vi "Gen - Button Disable.vi"(6 "State":enum16{"Enable", "Disable", "Disable & Gray"}(ring), 8 "Error In":errorcluster, 11 "Ref in":refnum<vi>) -> (0 "Error Out":errorcluster)   [LabVIEW 2020]
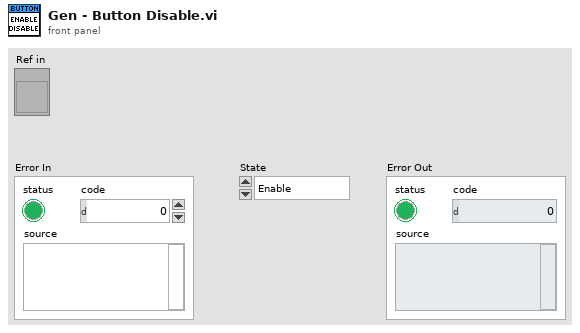
[diagram p1: front panel]
types:
  T1 = enum8{"Enabled", "Disabled", "Disabled and Grayed Out"}
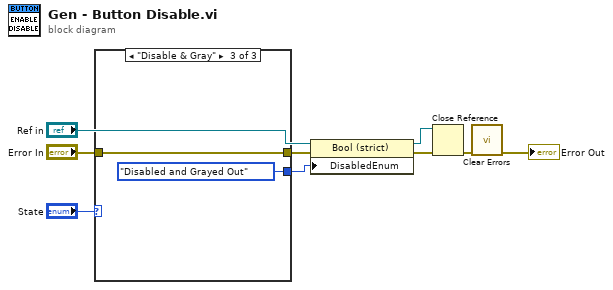
[diagram p0: block diagram]
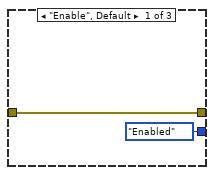
[diagram p2: hidden frame]
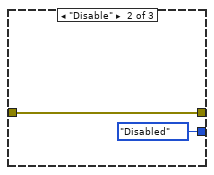
[diagram p3: hidden frame]
diagram:
  n1 = case shown="\"Disable & Gray\"" "State" {
    tunnel: [T1."Enabled" ("State") T1."Disabled" ("State") T1."Disabled and Grayed Out" ("State")] -> w1
    tunnel: [w11 w13 w15] -> w6
    tunnel: "Error In" -> [w11 w13 w15]
    frame "Enable", Default {
    }
    frame "Disable" {
    }
    frame "Disable & Gray" {
    }
  }
  n2 = property class="Bool (strict)"(reference="Ref in", error in=w6, "DisabledEnum"=w1) -> (reference out=w3:refnum<vi>, error out=w9:errorcluster)
  n3 = Close Reference(reference=w3, error in (no error)=w9) -> (error out=w8:errorcluster)
  n4 = call <vilib>:"Clear Errors.vi"("error in (no error)"=w8) -> ("error out"=→"Error Out":errorcluster)  [unwired: 5 in, 1 out]
